vi "subApplyAlamoutiCode.vi"(11 "Modulated Stream":cdb[](array[numeric])) -> (3 "Baseband Streams":cdb[][](array[numeric]))   [LabVIEW 2011]
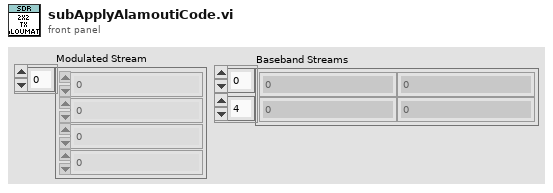
[diagram p1: front panel]
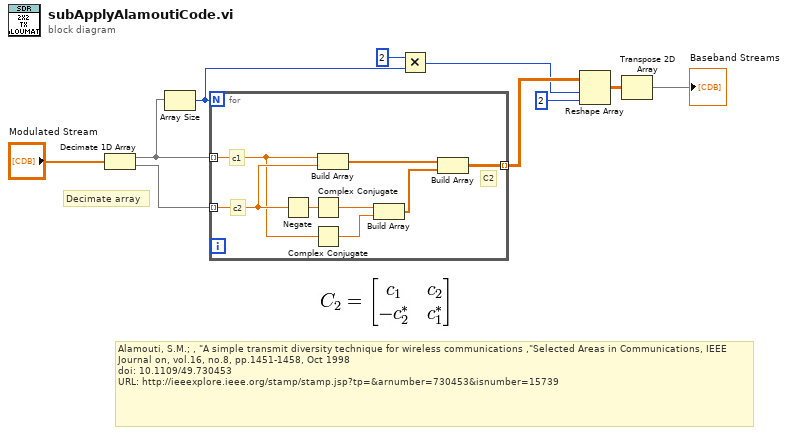
[diagram p0: block diagram]
diagram:
  # "Decimate array"
  # "Alamouti, S.M.; , \"A simple transmit diversity technique for wireless communications ,\"Selected Areas in Communications, IEEE Journal on, vol.16, no.8, pp.1451-1458, Oct 1998 \ndoi: 10.1109/49.730453\nURL: http://ieeexplore.ieee.org/stamp/stamp.jsp?tp=&arnumber=730453&isnumber=15739"
  n1 = Decimate 1D Array("Modulated Stream") -> (w9:cdb[], w10:cdb[])
  n2 = Array Size(array=w9) -> (size(s)=w3:i32)
  n3 = for {
    N: w3 -> [_]
    tunnel: w10 -> [w18] mode=indexing
    tunnel: w9 -> [w16] mode=indexing
    tunnel: [w13] -> w5 mode=indexing
    # "C2"
    # "c2"
    # "c1"
    n4 = Negate(x=w18) -> (-x=w17:cdb)
    n5 = Complex Conjugate(1:w17) -> (0:w15:cdb)
    n6 = Complex Conjugate(1:w16) -> (0:w14:cdb)
    n7 = Build Array(w16, w18) -> (w12:cdb[])
    n8 = Build Array(w15, w14) -> (w11:cdb[])
    n9 = Build Array(w12, w11) -> (w13:cdb[][])
  }
  n10 = Multiply(x=2, y=w3) -> (x*y=w2:i32)
  n11 = Reshape Array(w5, w2, 2 ("dimension size")) -> (w8:cdb[][])
  n12 = Transpose 2D Array(2D array=w8) -> (transposed array=→"Baseband Streams":cdb[][])
